vi "Estimate Absolute Orientation.vi"   [LabVIEW 2020, in "ar.lvlib"]
doc: "Estimate the Absolute Orientation of multiple views of the same 3D Point Set. \n\nThis can be used to combine multiple samples of the same object point sets to reduce mean square errors in an absolute set of positions."
uses:
  ar.lvlib
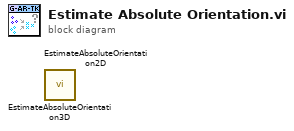
[diagram p0: block diagram]
diagram:
  n1 = call "EstimateAbsoluteOrientation3D.vi"() -> ()  [unwired: 7 in, 5 out]
  n2 = call "EstimateAbsoluteOrientation2D.vi"() -> ()  [unwired: 7 in, 5 out]
